vi "Start.vi"() -> ()   [LabVIEW 2016]
uses:
  <vilib>/Utility/miscctls.llb/LVPointTypeDef.ctl
panel:
  in  "Cancel Button":bool
  in  "OK Button":bool
  in  "Software Menu":i32(ring) caption="Software Configuration" items=["Oxford 4Pi soft", "Oxford 4Pi soft", "Oxford 4Pi soft_4piAbMode", "4piOxSoftCfg_focusLock", "Example Microscope", "User Select"]
  in  "Hardware Menu":i32(ring) caption="Hardware Configuration" items=["Oxford 4Pi hard", "Oxford 4Pi hard", "4Pi Microscope", "Example Microscope", "ObjLock_4PiHdCfg", "Ox4PiHardCfg_Win10.txt", "User Select"]
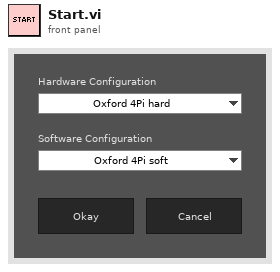
[diagram p1: front panel]
types:
  T1 = enum16{"Always On", "Always Off", "Off While Running"}
  T2 = typedef "LVPointTypeDef.ctl" = cluster{"Horizontal":i16, "Vertical":i16}
  T3 = enum32{"Invalid", "Standard", "Closed", "Hidden", "Minimized", "Maximized"}
  T4 = typedef "LVRectTypeDef.ctl" = cluster{"Left":i16, "Top":i16, "Right":i16, "Bottom":i16}
  T5 = typedef "LVBoundsTypeDef.ctl" = cluster{"Width":u32, "Height":u32}
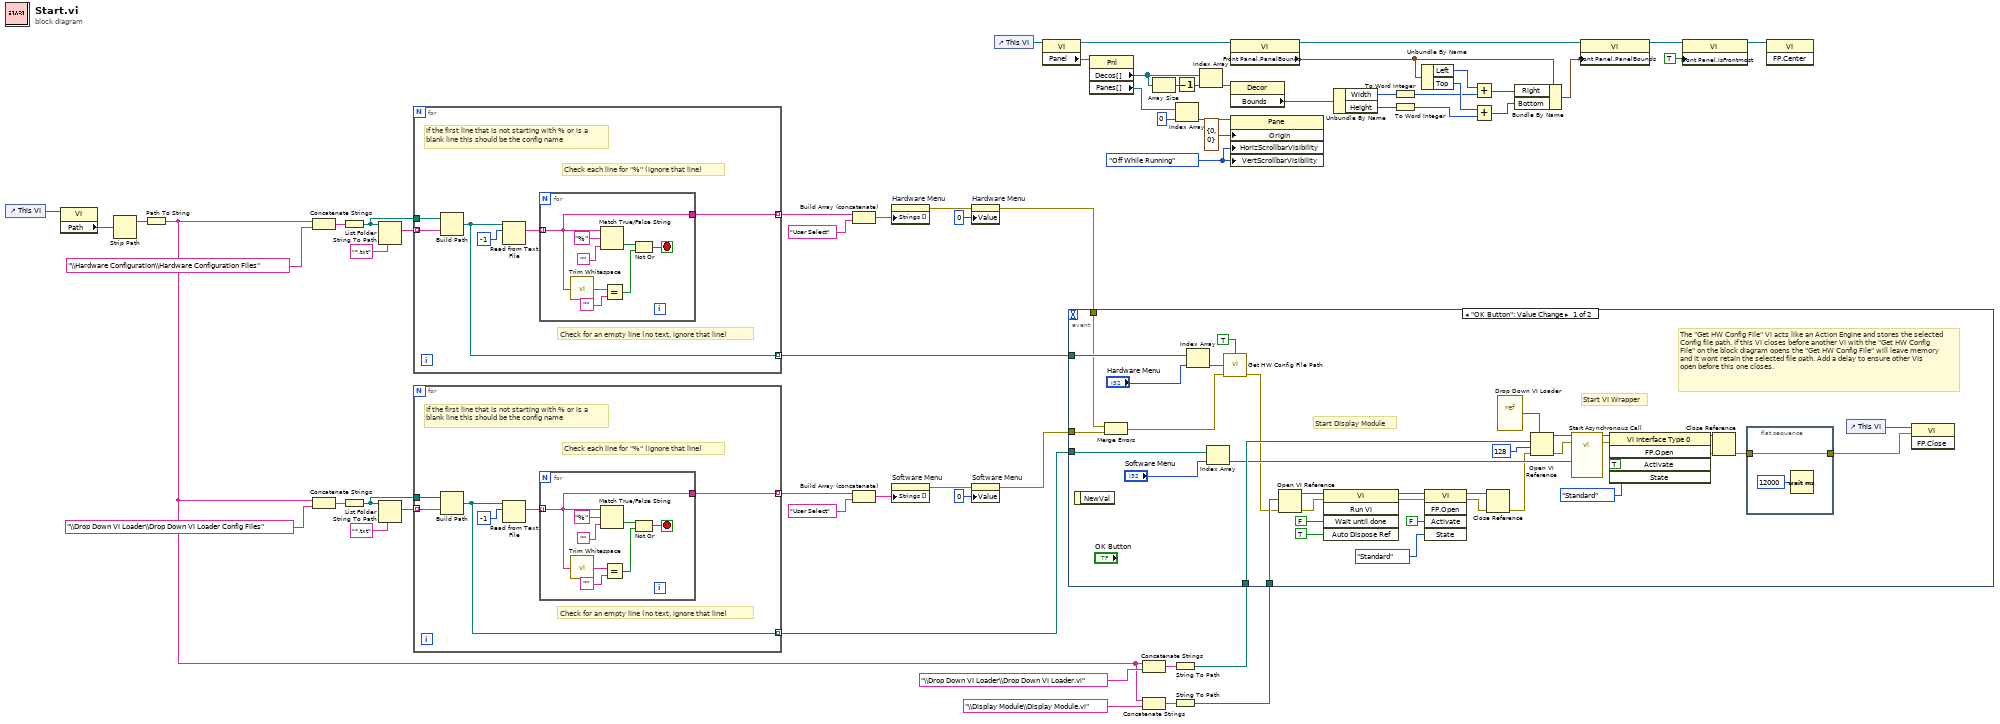
[diagram p0: block diagram]
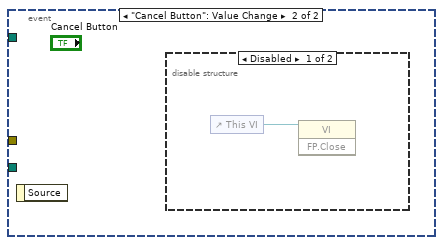
[diagram p2: hidden frame]
diagram:
  w15 = T1."Off While Running" ("Vertical Scrollbar Visibility")
  n1 = control-ref of="This VI"() -> (w61:refnum<vi>)
  n2 = property class="VI"(reference=w61) -> ("Path"=w60:path)  [unwired: 1 in, 2 out]
  n3 = Strip Path(path=w60) -> (stripped path=w59:path)  [unwired: 1 out]
  n4 = Path To String(path=w59) -> (string=w28:string)
  n5 = Concatenate Strings(w28, "\\Hardware Configuration\\Hardware Configuration Files") -> (w53:string)
  n6 = Concatenate Strings(w28, "\\Drop Down VI Loader\\Drop Down VI Loader Config Files") -> (w54:string)
  n7 = String To Path(string=w53) -> (path=w51:path)
  n8 = String To Path(string=w54) -> (path=w49:path)
  n9 = List Folder(path=w51, pattern="*.txt") -> (filenames=w52:string[])  [unwired: 2 in, 3 out]
  n10 = List Folder(path=w49, pattern="*.txt") -> (filenames=w50:string[])  [unwired: 2 in, 3 out]
  n11 = for {
    tunnel: w52 -> [w67] mode=indexing
    tunnel: w51 -> [w66]
    tunnel: [w63] -> w48 mode=indexing
    tunnel: [w62] -> w42 mode=indexing
    # "If the first line that is not starting with % or is a\nblank line this should be the config name"
    # "Check for an empty line (no text, ignore that line)"
    # "Check each line for \"%\" (ignore that line)"
    n12 = Build Path(base path=w66, name or relative path=w67) -> (appended path=w62:path)
    n13 = Read from Text File(file (use dialog)=w62, count=-1) -> (text=w65:string[])  [unwired: 2 in, 3 out]
    n14 = for {
      tunnel: w65 -> [w68] mode=indexing
      tunnel: [w68] -> w63
      stop <- w69 stop-if-true
      n15 = call <vilib>:"Trim Whitespace.vi"("string"=w68) -> ("trimmed string"=w73:string)  [unwired: 1 in]
      n16 = Match True/False String(2:"", 3:"%" ("true string"), 4:w68) -> (0:w71:bool)  [unwired: 1 out]
      n17 = Equal?(x=w73, y="") -> (x = y?=w70:bool)
      n18 = Not Or(1:w70, 2:w71) -> (0:w69:bool)
    }
  }
  n19 = for {
    tunnel: w50 -> [w81] mode=indexing
    tunnel: w49 -> [w80]
    tunnel: [w77] -> w46 mode=indexing
    tunnel: [w76] -> w41 mode=indexing
    # "If the first line that is not starting with % or is a\nblank line this should be the config name"
    # "Check for an empty line (no text, ignore that line)"
    # "Check each line for \"%\" (ignore that line)"
    n20 = Build Path(base path=w80, name or relative path=w81) -> (appended path=w76:path)
    n21 = Read from Text File(file (use dialog)=w76, count=-1) -> (text=w79:string[])  [unwired: 2 in, 3 out]
    n22 = for {
      tunnel: w79 -> [w82] mode=indexing
      tunnel: [w82] -> w77
      stop <- w83 stop-if-true
      n23 = call <vilib>:"Trim Whitespace.vi"("string"=w82) -> ("trimmed string"=w87:string)  [unwired: 1 in]
      n24 = Match True/False String(2:"", 3:"%" ("true string"), 4:w82) -> (0:w85:bool)  [unwired: 1 out]
      n25 = Equal?(x=w87, y="") -> (x = y?=w84:bool)
      n26 = Not Or(1:w84, 2:w85) -> (0:w83:bool)
    }
  }
  n27 = Build Array (concatenate)(w48, "User Select" ("string")) -> (w43:string[])
  n28 = Build Array (concatenate)(w46, "User Select" ("string")) -> (w44:string[])
  n29 = property on="Hardware Menu" class="Ring (strict)"("Strings []"=w43) -> (error out=w36:errorcluster)  [unwired: 2 in, 1 out]
  n30 = property on="Software Menu" class="Ring (strict)"("Strings []"=w44) -> (error out=w38:errorcluster)  [unwired: 2 in, 1 out]
  n31 = property on="Hardware Menu" class="Ring (strict)"(error in=w36, "Value"=0) -> (error out=w35:errorcluster)  [unwired: 1 in, 1 out]
  n32 = property on="Software Menu" class="Ring (strict)"(error in=w38, "Value"=0) -> (error out=w37:errorcluster)  [unwired: 1 in, 1 out]
  n33 = control-ref of="This VI"() -> (w8:refnum<vi>)
  n34 = property class="VI"(reference=w8) -> (reference out=w16:refnum<vi>, "Panel"=w9:refnum<vi>)  [unwired: 1 in, 1 out]
  n35 = property class="Pnl"(reference=w9) -> ("Decos[]"=w7:refnum<vi>[], "Panes[]"=w12:refnum<vi>[])  [unwired: 1 in, 2 out]
  n36 = Concatenate Strings(w28, "\\Drop Down VI Loader\\Drop Down VI Loader.vi") -> (w33:string)
  n37 = Concatenate Strings(w28, "\\Display Module\\Display Module.vi") -> (w31:string)
  n38 = Array Size(array=w7) -> (size(s)=w5:i32)
  n39 = String To Path(string=w33) -> (path=w32:path)
  n40 = String To Path(string=w31) -> (path=w29:path)
  n41 = event shown="[0] \"OK Button\": Value Change" {
    selector: _ -> [_ _]
    dyn-events: _ -> [_ _]
    timeout: _ -> [_ _]
    tunnel: w42 -> [w126 _]
    tunnel: w41 -> [w124 _]
    tunnel: w37 -> [w116 _]
    tunnel: w35 -> [w117 _]
    tunnel: w32 -> [w122 _]
    tunnel: w29 -> [w120 _]
    event "OK Button": Value Change {
      # "The \"Get HW Config File\" VI acts like an Action Engine and stores the selected Config file path. If this VI closes before another VI with the \"Get HW Config File\" on the block diagram opens the \"Get HW Config File\" will leave memory and it wont retain the selected file path. Add a delay to ensure other VIs open before this one closes."
      # "Start VI Wrapper"
      # "Start Display Module"
      n42 = event-data() -> ()  [unwired: 1 in, 1 out]
      n43 = Merge Errors(w117, w116) -> (w115:errorcluster)
      n44 = Index Array(array=w126, index="Hardware Menu") -> (element=w119:path)
      n45 = Index Array(array=w124, index="Software Menu") -> (element=w121:path)
      n46 = call "Get HW Config File Path.vi"("Reset/Set File Path (F)?"=TRUE, "File Path"=w119, "Error"=w115) -> ("Error"=w93:errorcluster)  [unwired: 11 in, 1 out]
      n47 = Open VI Reference(vi path=w120, error in (no error)=w93) -> (vi reference=w107:refnum<vi>, error out=w94:errorcluster)  [unwired: 4 in]
      n48 = invoke class="VI" method="Run VI"(reference=w107, error in=w94, "Wait until done"=FALSE ("Wait Until Done"), "Auto Dispose Ref"=TRUE ("Auto Dispose Reference")) -> (reference out=w104:refnum<vi>, error out=w95:errorcluster)  [unwired: 1 in, 3 out]
      n49 = invoke class="VI" method="FP.Open"(reference=w104, error in=w95, "Activate"=FALSE ("Activate?"), "State"=T3."Standard") -> (reference out=w101:refnum<vi>, error out=w96:errorcluster)  [unwired: 1 in, 3 out]
      n50 = Close Reference(reference=w101, error in (no error)=w96) -> (error out=w97:errorcluster)
      n51 = vi-ref "Drop Down VI Loader.vi"() -> (w113:refnum<vi>)
      n52 = Open VI Reference(type specifier VI Refnum (for type only)=w113, vi path=w122, options=128, error in (no error)=w97) -> (vi reference=w112:refnum<vi>, error out=w100:errorcluster)  [unwired: 2 in]
      n53 = call-by-ref "Start Asynchronous Call"(reference=w112, error in=w100, "Software Config File Path"=w121) -> (reference out=w111:refnum<vi>, error out=w99:errorcluster)  [unwired: 15 in]
      n54 = invoke class="VI Interface Type 0" method="FP.Open"(reference=w111, error in=w99, "Activate"=TRUE ("Activate?"), "State"=T3."Standard") -> (reference out=w108:refnum<vi>, error out=w98:errorcluster)  [unwired: 1 in, 3 out]
      n55 = Close Reference(reference=w108, error in (no error)=w98) -> (error out=w92:errorcluster)
      n56 = flat-sequence {
        tunnel: w92 -> [w127]
        tunnel: [w127] -> w90
        frame #0 {
          n57 = Wait (ms)(milliseconds to wait=u32 12000) -> ()  [unwired: 1 out]
        }
      }
      n58 = control-ref of="This VI"() -> (w91:refnum<vi>)
      n59 = invoke class="VI" method="FP.Close"(reference=w91, error in=w90) -> ()  [unwired: 1 in, 3 out]
    }
    event "Cancel Button": Value Change {
      n60 = event-data() -> ()  [unwired: 1 in, 1 out]
      n61 = disable-structure shown="Disabled" {
        frame Disabled {
          n62 = control-ref of="This VI"() -> (w129:refnum<vi>)
          n63 = invoke class="VI" method="FP.Close"(reference=w129) -> ()  [unwired: 2 in, 3 out]
        }
        frame Enabled {
        }
      }
    }
  }
  n64 = Decrement(x=w5) -> (x-1=w6:i32)
  n65 = Index Array(array=w12, index=0) -> (element=w11:refnum<vi>)
  n66 = Index Array(array=w7, index=w6) -> (element=w14:refnum<vi>)
  n67 = property class="VI"(reference=w16) -> (reference out=w18:refnum<vi>, "Front Panel.PanelBounds"=w19:T4)  [unwired: 1 in, 1 out]
  n68 = property class="Decor"(reference=w14) -> ("Bounds"=w17:T5)  [unwired: 1 in, 2 out]
  n69 = property class="Pane"(reference=w11, "Origin"=T2 {"Horizontal"=0, "Vertical"=0}, "HorizScrollbarVisibility"=w15, "VertScrollbarVisibility"=w15) -> ()  [unwired: 1 in, 2 out]
  n70 = Unbundle By Name(w17) -> ("Width"=w22:u32, "Height"=w25:u32)
  n71 = To Word Integer(number=w22) -> (16bit integer=w24:i16)
  n72 = To Word Integer(number=w25) -> (16bit integer=w4:i16)
  n73 = Unbundle By Name(w19) -> ("Left"=w21:i16, "Top"=w27:i16)
  n74 = Add(x=w21, y=w24) -> (x+y=w23:i16)
  n75 = Add(x=w27, y=w4) -> (x+y=w26:i16)
  n76 = Bundle By Name(cluster=w19, "Right"=w23, "Bottom"=w26) -> (w20:T4)
  n77 = property class="VI"(reference=w18, "Front Panel.PanelBounds"=w20) -> (reference out=w3:refnum<vi>)  [unwired: 1 in, 1 out]
  n78 = property class="VI"(reference=w3, "Front Panel.IsFrontmost"=TRUE ("Front Panel Window:Is Frontmost")) -> (reference out=w1:refnum<vi>)  [unwired: 1 in, 1 out]
  n79 = invoke class="VI" method="FP.Center"(reference=w1) -> ()  [unwired: 2 in, 3 out]
